vi "RawRegistry.vi"(8 "error in (no error)":errorcluster, 11 "navX - Base in":refnum<class "navX - Base.lvclass">) -> (0 "error out":errorcluster, 2 "Registry Cache out":u8[](array[numeric]), 3 "navX - Base out":refnum<class "navX - Base.lvclass">)   [LabVIEW 2015, in "navX Library v3.lvlib" / "navX - Base.lvclass"]
uses:
  navX - Base.lvclass
  navX - Base.lvclass/navX - Base.ctl
  navX Registry Cache/navX Registry Cache.lvclass
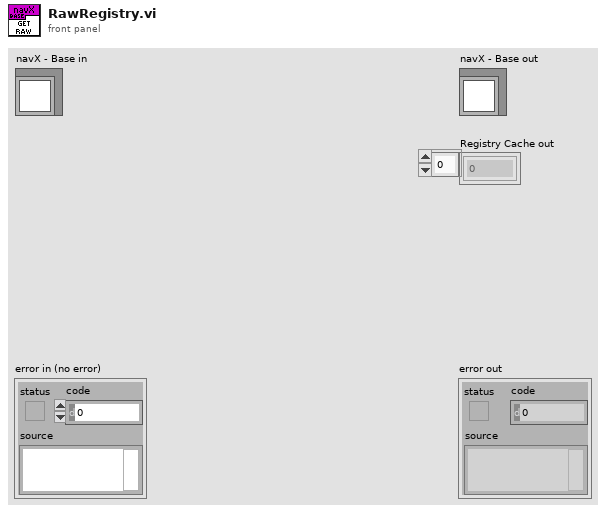
[diagram p1: front panel]
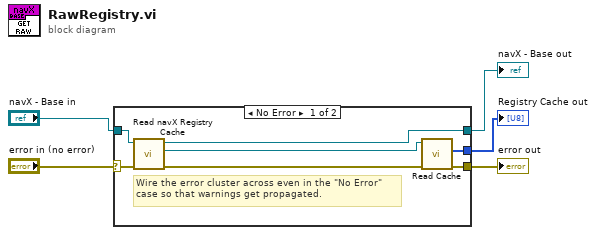
[diagram p0: block diagram]
diagram:
  n1 = case shown="No Error" "error in (no error)" {
    selector: "error in (no error)" -> [w8 w14]
    tunnel: [w7 w14] -> w4
    tunnel: [w6 w13] -> w2
    tunnel: "navX - Base in" -> [w12 w13]
    tunnel: [w9 _] -> w1
    frame No Error {
      # "Wire the error cluster across even in the \"No Error\"\ncase so that warnings get propagated."
      n2 = call "Read navX Registry Cache.vi"("error in (no error)"=w8, "navX - Base in"=w12) -> ("error out"=w10:errorcluster, "navX Library v3.lvlib:navX Registry Cache.lvclass"=w11:refnum<class "navX Registry Cache.lvclass">, "navX - Base out"=w6:refnum<class "navX - Base.lvclass">)  [unwired: 7 in]
      n3 = call "Read Cache.vi"("error in (no error)"=w10, "navX Registry Cache in"=w11) -> ("error out"=w7:errorcluster, "Registry Cache out"=w9:u8[])  [unwired: 7 in, 1 out]
    }
    frame Error {
    }
  }
  "error out" <- w4
  "navX - Base out" <- w2
  "Registry Cache out" <- w1
